vi "SGUI Example - demo 2.vi"() -> ()   [LabVIEW 2020, in "varilib.lvlib"]
doc: "SGUI lib demo 2. Demonstration of control groups usage and controling controls from different VI."
uses:
  varilib.lvlib
  SGUI Assign References Mode.ctl
panel:
  in  "btn sub-panel":bool
  out "error out":errorcluster
  in  "btn exit":bool
  out "my int32":i32
  in  "btn stop":bool
  in  "btn start":bool
  in  "N":i32
  # "group 'ready'"
  # "group 'busy'"
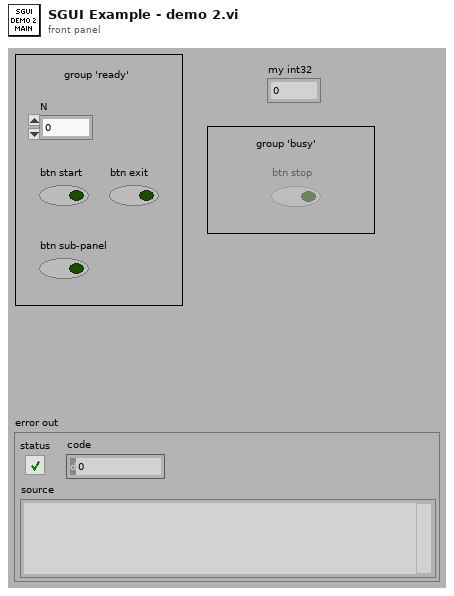
[diagram p1: front panel]
types:
  T1 = typedef "varilib.lvlib/SGUI Assign References Mode.ctl" = enum16{"Add to stack", "Overwrite", "Release last", "Release ID"}
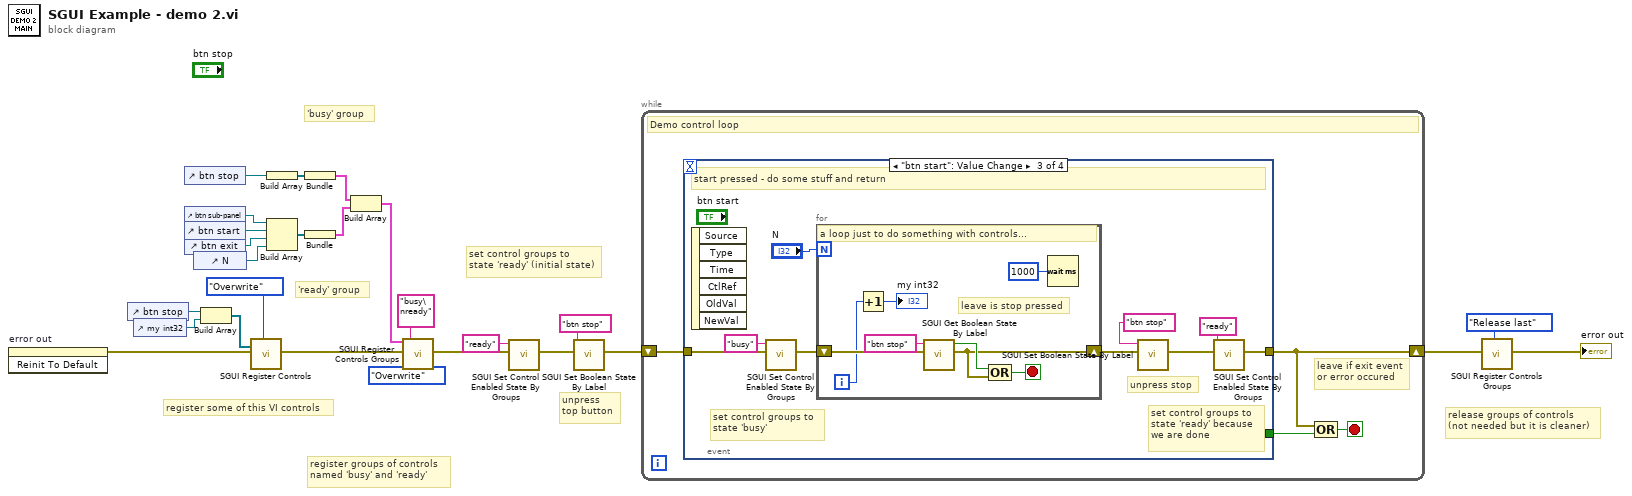
[diagram p0: block diagram]
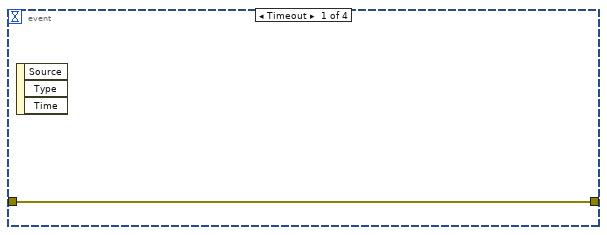
[diagram p2: hidden frame]
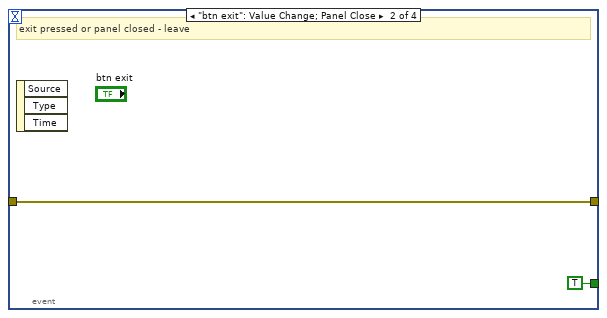
[diagram p3: hidden frame]
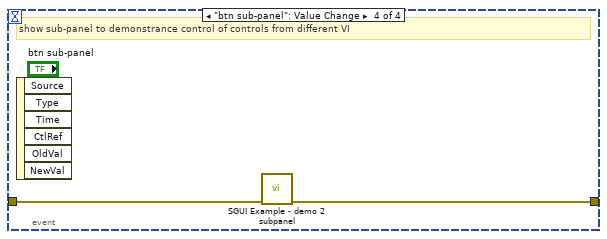
[diagram p4: hidden frame]
diagram:
  # "'ready' group"
  # "'busy' group"
  # "set control groups to\nstate 'ready' (initial state)"
  # "release groups of controls\n(not needed but it is cleaner)"
  # "unpress\ntop button"
  # "register groups of controls\nnamed 'busy' and 'ready'"
  # "register some of this VI controls"
  n1 = invoke on="error out" class="Clust (strict)" method="Reinit To Default"() -> (error out=w8:errorcluster)  [unwired: 3 in, 2 out]
  n2 = control-ref of="btn stop"() -> (w25:refnum<vi>)
  n3 = control-ref of="my int32"() -> (w1:refnum<vi>)
  n4 = control-ref of="btn stop"() -> (w20:refnum<vi>)
  n5 = control-ref of="btn sub-panel"() -> (w2:refnum<vi>)
  n6 = control-ref of="btn start"() -> (w22:refnum<vi>)
  n7 = control-ref of="btn exit"() -> (w21:refnum<vi>)
  n8 = control-ref of="N"() -> (w12:refnum<vi>)
  n9 = Build Array(w25, w1) -> (w24:refnum<vi>[])
  n10 = call "SGUI Register Controls.vi"("error in"=w8, "control references (empty)"=w24, "register mode (overwrite)"=SGUI_Assign_References_Mode."Overwrite") -> ("error out"=w26:errorcluster)  [unwired: 14 in, 2 out]
  n11 = Build Array(w20) -> (w19:refnum<vi>[])
  n12 = Build Array(w2, w22, w21, w12) -> (w18:refnum<vi>[])
  n13 = Bundle(w19) -> (w17:cluster{refnum<vi>[]})  [unwired: 1 in]
  n14 = Bundle(w18) -> (w16:cluster{refnum<vi>[]})  [unwired: 1 in]
  n15 = Build Array(w17, w16) -> (w15:cluster{refnum<vi>[]}[])
  n16 = call "SGUI Register Controls Groups.vi"("control groups"=w15, "error in"=w26, "groups names"="busy\nready", "register mode (overwrite)"=SGUI_Assign_References_Mode."Overwrite") -> ("error out"=w4:errorcluster)  [unwired: 14 in, 1 out]
  n17 = call "SGUI Set Control Enabled State By Groups.vi"("error in"=w4, "group name to enable (none)"="ready") -> ("error out"=w3:errorcluster)  [unwired: 8 in, 1 out]
  n18 = call "SGUI Set Boolean State By Label.vi"("error in"=w3, "control label(s) ('btn stop')"="btn stop" ("control label ('btn stop')")) -> ("error out"=w7:errorcluster)  [unwired: 8 in, 1 out]
  n19 = while {
    shift-right: [w27] -> w11
    shift-left: w7 -> [w30]
    stop <- w29 stop-if-true
    # "leave if exit event\nor error occured"
    # "Demo control loop"
    n20 = event shown="[2] \"btn start\": Value Change" {
      selector: _ -> [_ _ _ _]
      dyn-events: _ -> [_ _ _ _]
      timeout: _ -> [_ _ _ _]
      tunnel: w30 -> [w31 w33 w42 w52]
      tunnel: [w31 w33 w38 w51] -> w27
      tunnel: [_ TRUE _ _] -> w28
      event Timeout {
        n21 = event-data() -> ()  [unwired: 1 in, 3 out]
      }
      event "btn exit": Value Change; Panel Close {
        # "exit pressed or panel closed - leave"
        n22 = event-data() -> ()  [unwired: 1 in, 3 out]
      }
      event "btn start": Value Change {
        # "unpress stop"
        # "set control groups to\nstate 'ready' because \nwe are done"
        # "set control groups to\nstate 'busy'"
        # "start pressed - do some stuff and return"
        n23 = event-data() -> ()  [unwired: 1 in, 6 out]
        n24 = call "SGUI Set Control Enabled State By Groups.vi"("error in"=w42, "group name to enable (none)"="busy") -> ("error out"=w41:errorcluster)  [unwired: 8 in, 1 out]
        n25 = for {
          N: "N" -> [_]
          shift-right: [w46] -> w36
          shift-left: w41 -> [w50]
          i -> [w45]
          stop <- w48 stop-if-true
          # "leave is stop pressed"
          # "a loop just to do something with controls..."
          n26 = Increment(x=w45) -> (x+1=→"my int32":i32)
          n27 = call "SGUI Get Boolean State By Label.vi"("error in"=w50, "control label ('btn stop')"="btn stop") -> ("error out"=w46:errorcluster, "binary state out"=w47:bool)  [unwired: 7 in, 1 out]
          n28 = Compound Arithmetic op=OR(w47, w46) -> (w48:bool)
          n29 = Wait (ms)(milliseconds to wait=u32 1000) -> ()  [unwired: 1 out]
        }
        n30 = call "SGUI Set Boolean State By Label.vi"("error in"=w36, "control label(s) ('btn stop')"="btn stop" ("control label ('btn stop')")) -> ("error out"=w35:errorcluster)  [unwired: 8 in, 1 out]
        n31 = call "SGUI Set Control Enabled State By Groups.vi"("error in"=w35, "group name to enable (none)"="ready") -> ("error out"=w38:errorcluster)  [unwired: 8 in, 1 out]
      }
      event "btn sub-panel": Value Change {
        # "show sub-panel to demonstrance control of controls from different VI"
        n32 = event-data() -> ()  [unwired: 1 in, 6 out]
        n33 = call "SGUI Example - demo 2 subpanel.vi"("error in (no error)"=w52) -> ("error out"=w51:errorcluster)  [unwired: 10 in]
      }
    }
    n34 = Compound Arithmetic op=OR(w27, w28) -> (w29:bool)
  }
  n35 = call "SGUI Register Controls Groups.vi"("error in"=w11, "register mode (overwrite)"=SGUI_Assign_References_Mode."Release last") -> ("error out"=→"error out":errorcluster)  [unwired: 16 in, 1 out]
